vi "Query Status.vi"(8 "error in (no error)":errorcluster, 10 "Address (1)":u16=1 max=15 step=1, 11 "VISA resource name":refnum<visa-resource-name>) -> (0 "error out":errorcluster, 2 "Status":bool, 3 "VISA resource name out":refnum<visa-resource-name>)   [LabVIEW 2021, in "Copy of Kloehn V6 Series.lvlib"]
doc: "Queries the instrument for its current status. It will either be busy doing some operation or ready to receive an operation to carry out."
uses:
  Copy of Kloehn V6 Series.lvlib
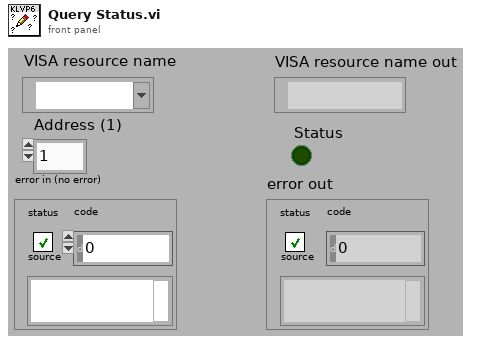
[diagram p1: front panel]
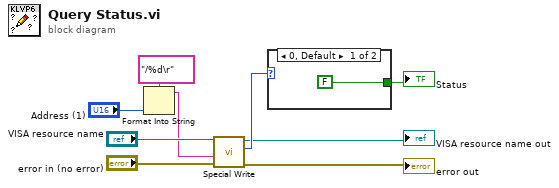
[diagram p0: block diagram]
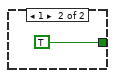
[diagram p2: hidden frame]
diagram:
  n1 = Format Into String(format string="/%d\r", "Address (1)") -> (resulting string=w5:string)  [unwired: 2 in, 1 out]
  n2 = call "Special Write.vi"("error in (no error)"="error in (no error)", "Send String"=w5, "VISA resource name"="VISA resource name") -> ("error out"=→"error out":errorcluster, "Status"=w2:u16, "VISA resource name out"=→"VISA resource name out":refnum<visa-resource-name>)  [unwired: 4 in, 2 out]
  n3 = case shown="0, Default" w2 {
    tunnel: [FALSE TRUE] -> w7
    frame 0, Default {
    }
    frame 1 {
    }
  }
  "Status" <- w7
